vi "main.vi"() -> ()   [LabVIEW 2018]
doc: "Main application window for the adaSuite home automation system. This VI should serve as the main launching point for changing system information, accessing sensor probes, creating dashboards; etc."
uses:
  <vilib>/Utility/config.llb/Read Key (Boolean).vi
  <vilib>/Utility/config.llb/Read Key (String).vi
  <vilib>/Utility/config.llb/Write Key (Boolean).vi
  <vilib>/Utility/config.llb/Write Key (String).vi
  <vilib>/Utility/config.llb/NI_LVConfig.lvlib
panel:
  in  "Boolean":bool
  in  "Quit Button":bool
  out "error out":errorcluster
  out "Address":string
  out "Dev Mode":bool
  in  "type specifier VI Refnum (for type only) 2":refnum<vi>
  # "wetter"
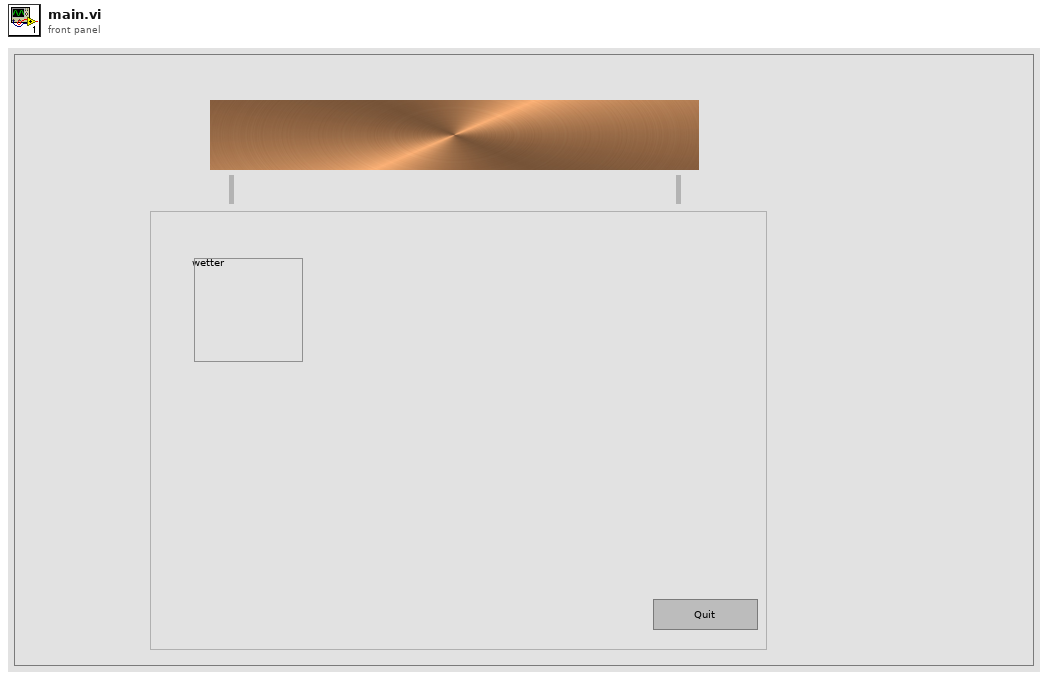
[diagram p1: front panel]
types:
  T1 = typedef "NI_LVConfig.lvlib/Config Data RefNum.ctl" = refnum<k1>
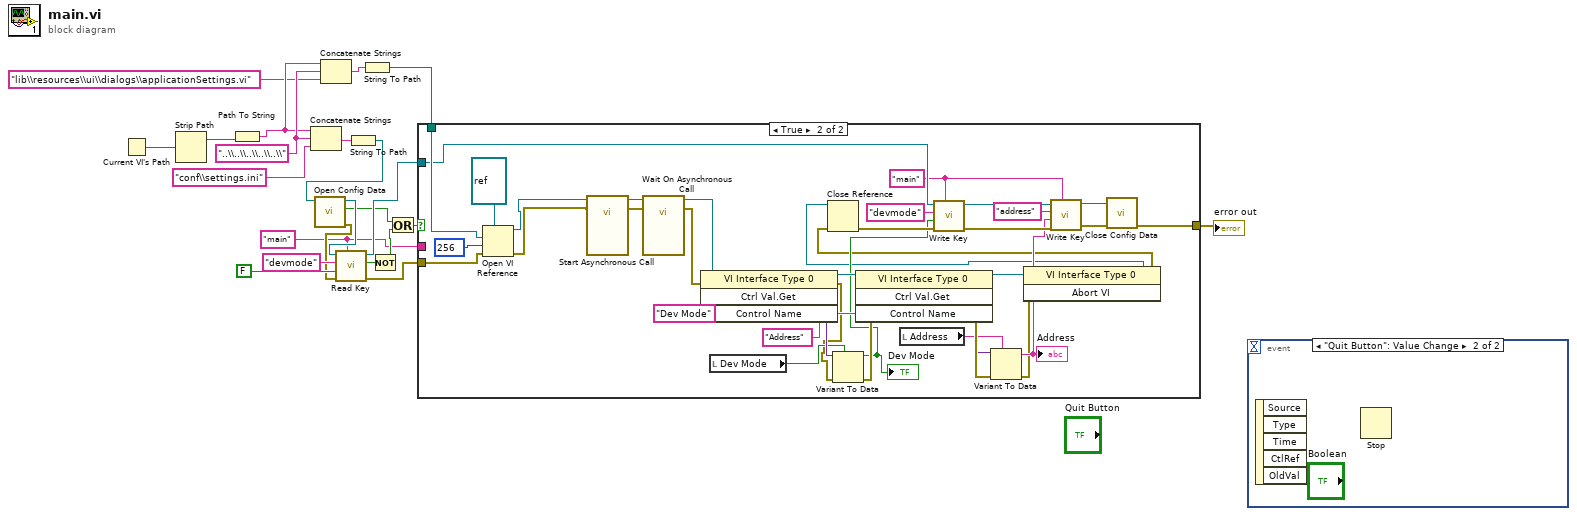
[diagram p0: block diagram]
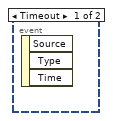
[diagram p2: hidden frame]
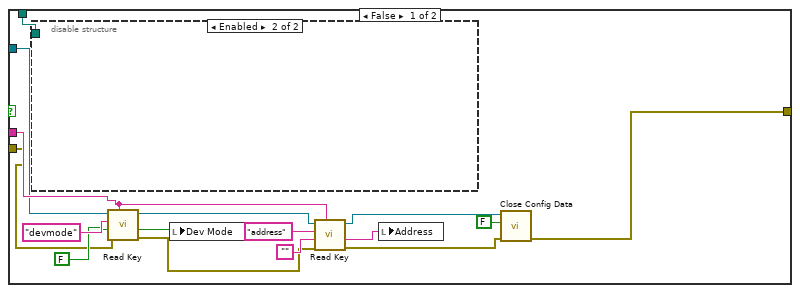
[diagram p3: hidden frame]
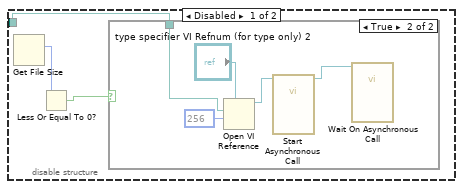
[diagram p4: hidden frame]
diagram:
  w1 = "main" ("section")
  w18 = "..\\..\\..\\..\\..\\"
  n1 = Current VI's Path() -> (path=w22:path)
  n2 = Strip Path(path=w22) -> (stripped path=w21:path)  [unwired: 1 out]
  n3 = Path To String(path=w21) -> (string=w17:string)
  n4 = Concatenate Strings(w17, w18, "conf\\settings.ini") -> (w20:string)
  n5 = Concatenate Strings(w17, w18, "lib\\resources\\ui\\dialogs\\applicationSettings.vi" ("string")) -> (w15:string)
  n6 = String To Path(string=w20) -> (path=w13:path)
  n7 = call <vilib>:"Open Config Data.vi"("configuration file path"=w13) -> ("error out"=w7:errorcluster, "file created?"=w3:bool, "refnum"=w11:T1)  [unwired: 8 in]
  n8 = call-poly <vilib>:"Read Key.vi"("section"=w1, "error in (no error)"=w7, "default value"=FALSE, "key"="devmode", "refnum"=w11) -> ("error out"=w6:errorcluster, "found?"=w5:bool, "refnum out"=w10:T1)  [unwired: 3 in, 1 out]
  n9 = String To Path(string=w15) -> (path=w14:path)
  n10 = Not(x=w5) -> (.not. x?=w4:bool)
  n11 = Or(x=w3, y=w4) -> (x .or. y?=w2:bool)
  n12 = case shown="True" w2 {
    tunnel: w14 -> [w38 w81]
    tunnel: w10 -> [w31 w79]
    tunnel: w6 -> [w32 w80]
    tunnel: [w23 w58] -> w12
    tunnel: w1 -> [w37 _]
    frame False {
      n13 = disable-structure shown="Enabled" {
        disable-tunnel: w38 -> [w40 _]
        frame Disabled {
          n14 = Get File Size() -> (size (in bytes)=w41:i64)  [unwired: 2 in, 2 out]
          n15 = Less Or Equal To 0?(x=w41) -> (x <= 0?=w39:bool)
          n16 = case shown="True" w39 {
            tunnel: w40 -> [_ w43]
            frame False {
            }
            frame True {
              n17 = Open VI Reference(type specifier VI Refnum (for type only)="type specifier VI Refnum (for type only) 2", vi path=w43, options=256) -> (vi reference=w45:refnum<vi>)  [unwired: 3 in, 1 out]
              n18 = call-by-ref "Start Asynchronous Call"(reference=w45) -> (reference out=w42:refnum<vi>)  [unwired: 13 in, 1 out]
              n19 = call-by-ref "Wait On Asynchronous Call"(reference=w42) -> ()  [unwired: 13 in, 2 out]
            }
          }
        }
        frame Enabled {
        }
      }
      n20 = call-poly <vilib>:"Read Key.vi"("section"=w37, "error in (no error)"=w32, "default value"=FALSE, "key"="devmode", "refnum"=w31) -> ("error out"=w30:errorcluster, "value"=w28:bool, "refnum out"=w29:T1)  [unwired: 3 in, 1 out]
      n21 = local write "Dev Mode"(w28) -> ()
      n22 = call-poly <vilib>:"Read Key.vi"("section"=w37, "error in (no error)"=w30, "default value"="", "key"="address", "refnum"=w29) -> ("error out"=w26:errorcluster, "value"=w27:string, "refnum out"=w25:T1)  [unwired: 3 in, 1 out]
      n23 = local write "Address"(w27) -> ()
      n24 = call <vilib>:"Close Config Data.vi"("error in (no error)"=w26, "write file if changed (T)"=FALSE, "refnum"=w25) -> ("error out"=w23:errorcluster)  [unwired: 7 in, 1 out]
    }
    frame True {
      w61 = "main" ("section")
      n25 = Open VI Reference(type specifier VI Refnum (for type only)=refnum<vi> refnum, vi path=w81, options=256, error in (no error)=w80) -> (vi reference=w47:refnum<vi>, error out=w48:errorcluster)  [unwired: 2 in]
      n26 = call-by-ref "Start Asynchronous Call"(reference=w47, error in=w48) -> (reference out=w52:refnum<vi>, error out=w49:errorcluster)  [unwired: 12 in]
      n27 = call-by-ref "Wait On Asynchronous Call"(reference=w52, error in=w49) -> (reference out=w51:refnum<vi>, error out=w50:errorcluster)  [unwired: 12 in]
      n28 = invoke class="VI Interface Type 0" method="Ctrl Val.Get"(reference=w51, error in=w50, "Control Name"="Dev Mode") -> (reference out=w75:refnum<vi>, error out=w71:errorcluster, "Get Control Value Variant"=w73:variant)  [unwired: 1 in, 1 out]
      n29 = local read "Dev Mode"() -> (w72:bool)
      n30 = Variant To Data(error in=w71, type=w72, Variant=w73) -> (data=w66:bool, error out=w70:errorcluster)
      "Dev Mode" <- w66
      n31 = invoke class="VI Interface Type 0" method="Ctrl Val.Get"(reference=w75, error in=w70, "Control Name"="Address") -> (reference out=w55:refnum<vi>, error out=w69:errorcluster, "Get Control Value Variant"=w68:variant)  [unwired: 1 in, 1 out]
      n32 = local read "Address"() -> (w67:string)
      n33 = Variant To Data(error in=w69, type=w67, Variant=w68) -> (data=w59:string, error out=w56:errorcluster)
      "Address" <- w59
      n34 = invoke class="VI Interface Type 0" method="Abort VI"(reference=w55, error in=w56) -> (reference out=w53:refnum<vi>, error out=w54:errorcluster)  [unwired: 1 in, 1 out]
      n35 = Close Reference(reference=w53, error in (no error)=w54) -> (error out=w78:errorcluster)
      n36 = call-poly <vilib>:"Write Key.vi"("section"=w61, "error in (no error)"=w78, "value"=w66, "key"="devmode", "refnum"=w79) -> ("error out"=w65:errorcluster, "refnum out"=w64:T1)  [unwired: 4 in, 1 out]
      n37 = call-poly <vilib>:"Write Key.vi"("section"=w61, "error in (no error)"=w65, "value"=w59, "key"="address", "refnum"=w64) -> ("error out"=w63:errorcluster, "refnum out"=w62:T1)  [unwired: 4 in, 1 out]
      n38 = call <vilib>:"Close Config Data.vi"("error in (no error)"=w63, "refnum"=w62) -> ("error out"=w58:errorcluster)  [unwired: 8 in, 1 out]
    }
  }
  "error out" <- w12
  n39 = event shown="[1] \"Quit Button\": Value Change" {
    selector: _ -> [_ _]
    dyn-events: _ -> [_ _]
    timeout: _ -> [_ _]
    event Timeout {
      n40 = event-data() -> ()  [unwired: 1 in, 3 out]
    }
    event "Quit Button": Value Change {
      n41 = event-data() -> ()  [unwired: 1 in, 5 out]
      n42 = Stop() -> ()  [unwired: 1 in]
    }
  }
